vi "MessageName.vi"(11 "PB Msg Template in":refnum<class "Msg.lvclass">) -> (2 "MessageName":string)   [LabVIEW 2020, in "ReplyOneDouble.lvlib" / "Msg.lvclass"]
uses:
  Msg.lvclass
  Msg.lvclass/Msg.ctl
  ReplyOneDouble.lvlib
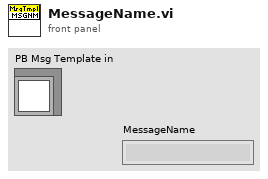
[diagram p1: front panel]
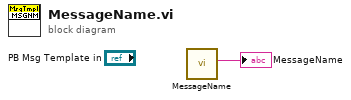
[diagram p0: block diagram]
diagram:
  n1 = call "MessageName.vi"() -> ("MessageName"=→"MessageName":string)  [unwired: 11 in]
